vi "EVT Camera Set U Int32Param.vi"(9 "val":u32, 10 "name":string, 11 "camera":u64) -> (3 "function return":u32(ring))   [LabVIEW 2019, in "EmergentCameraC.lvlib"]
doc: "EMERGENTCAMERAC_API EVT_ERROR EVT_CameraSetUInt32Param(Camera_Handle camera, const char* name, unsigned int val);"
uses:
  EmergentCameraC.lvlib
  emergentInstall_Windows/win64/eSDK/bin/EmergentCameraC.dll
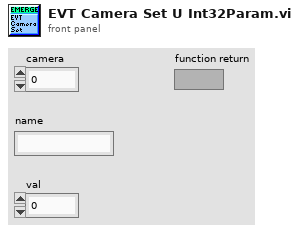
[diagram p1: front panel]
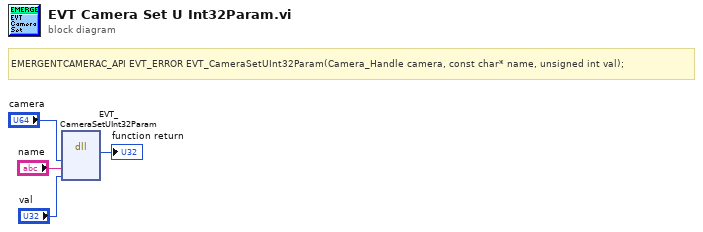
[diagram p0: block diagram]
diagram:
  # "EMERGENTCAMERAC_API EVT_ERROR EVT_CameraSetUInt32Param(Camera_Handle camera, const char* name, unsigned int val);"
  n1 = dll-call lib="E:/emergent/host-new_QT/emergentInstall_Windows/win64/eSDK/bin/EmergentCameraC.*" fn="EVT_CameraSetUInt32Param"("camera"="camera", "name"="name", "val"="val") -> (→"function return":u32)  [unwired: 6 in, 2 out]
